vi "TEST LVOOP Plug Ins - Solution.vi"(8 "error in (no error)":errorcluster, 10 "Queue Name":string="Main") -> (0 "error out":errorcluster)   [LabVIEW 2011]
doc: "This is the solution that for the LVOOP Plug Ins exercise. It illustrates the power and flexibility of LVOOP plug ins.\n\nAAL 9/09"
uses:
  Report Class/Report.lvclass
  Shared/QDMH Poly VIs/QDMH POLY Enqueue String.vi
  Shared/QDMH Poly VIs/QDMH POLY Enqueue Strings.vi
panel:
  in  "Get Plug Ins":bool
  in  "File Name (no extension)":string
  in  "Header":string
  in  "Save to File":bool
  in  "Available Plug Ins":u16(ring) items=["TXT Report", "XML Report"]
  out "Message Display":string
  in  "Cancel":bool
  in  "OK":bool
  # "You must specify file name above."
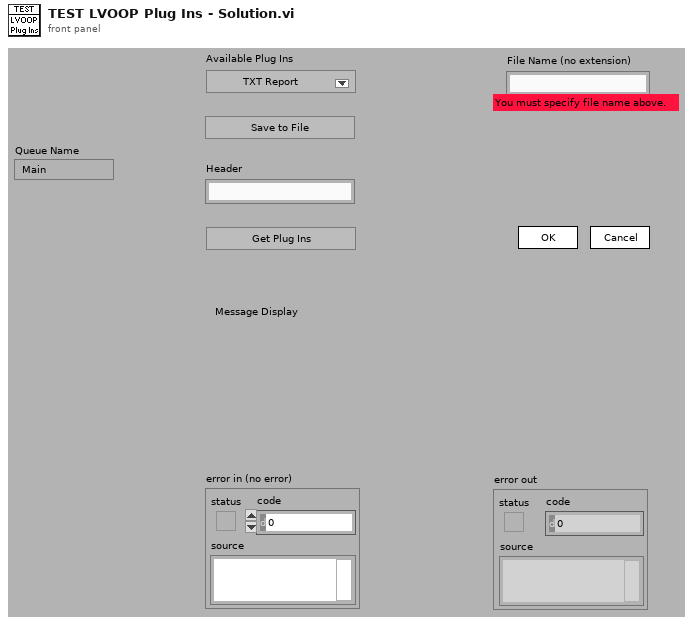
[diagram p1: front panel]
types:
  T1 = cluster{"Operator Name":string, "Current VI's Path":path, "Queue Names":string[], "# VIs Launched":i32, "Report Objects":refnum<class "Report.lvclass">[], "Selected Plug In":i32, "Current VI's Directory":path}
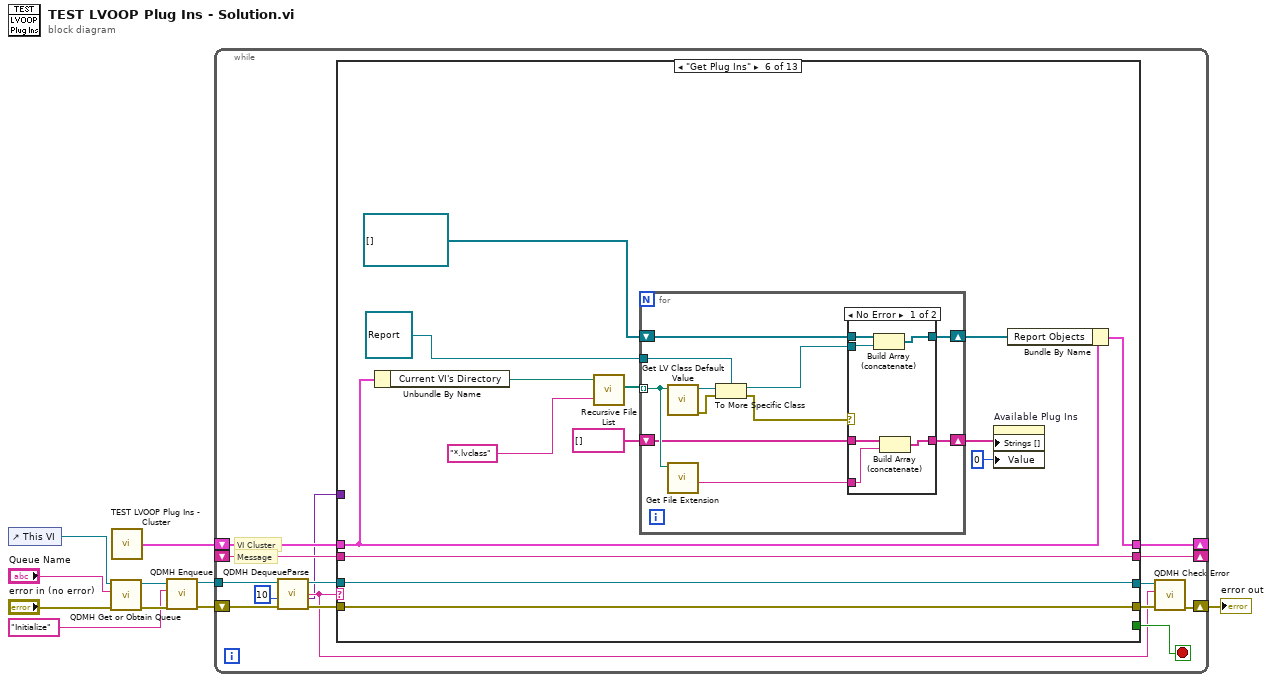
[diagram p0: block diagram]
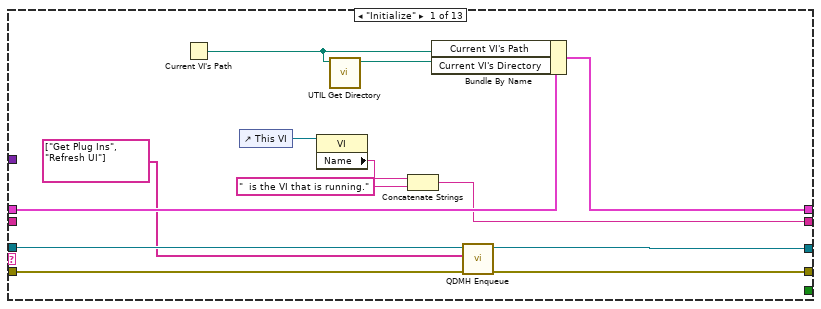
[diagram p2: hidden frame]
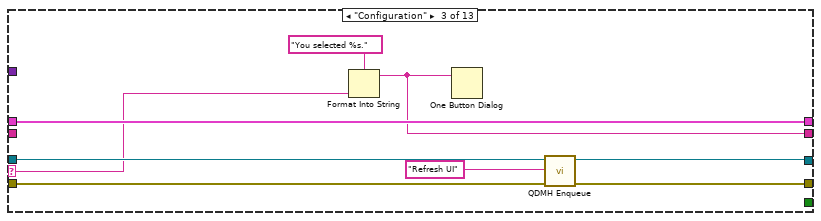
[diagram p4: hidden frame]
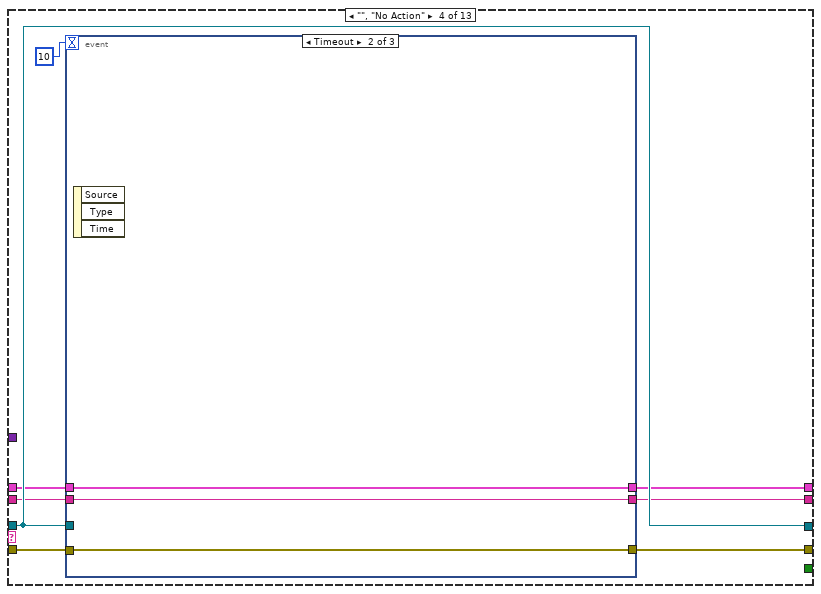
[diagram p5: hidden frame]
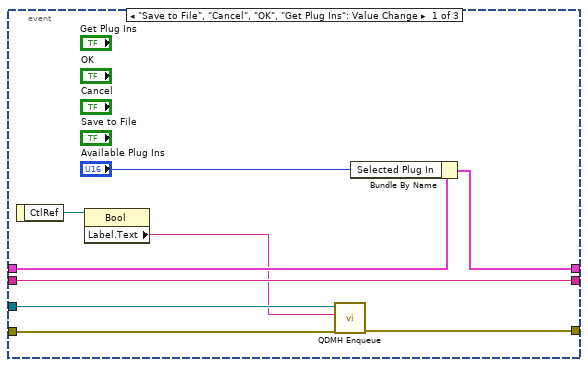
[diagram p6: hidden frame]
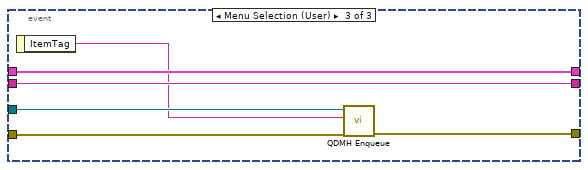
[diagram p7: hidden frame]
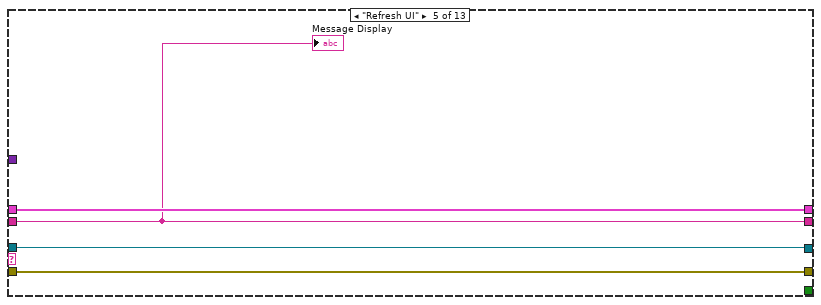
[diagram p8: hidden frame]
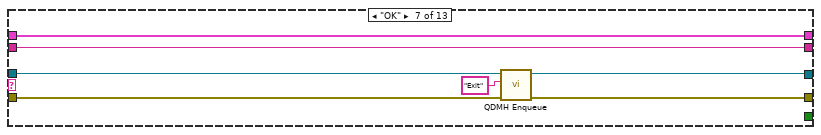
[diagram p10: hidden frame]
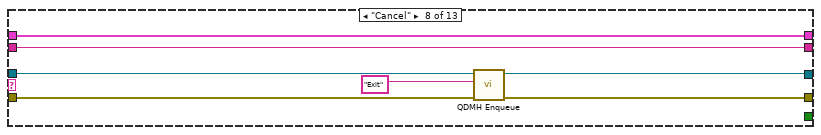
[diagram p11: hidden frame]
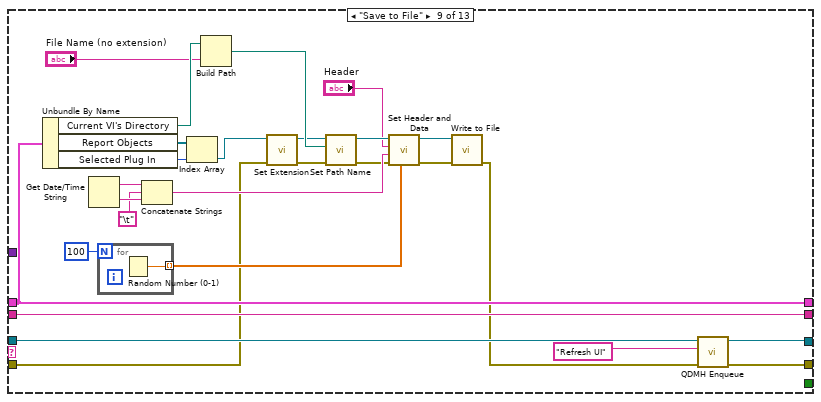
[diagram p12: hidden frame]
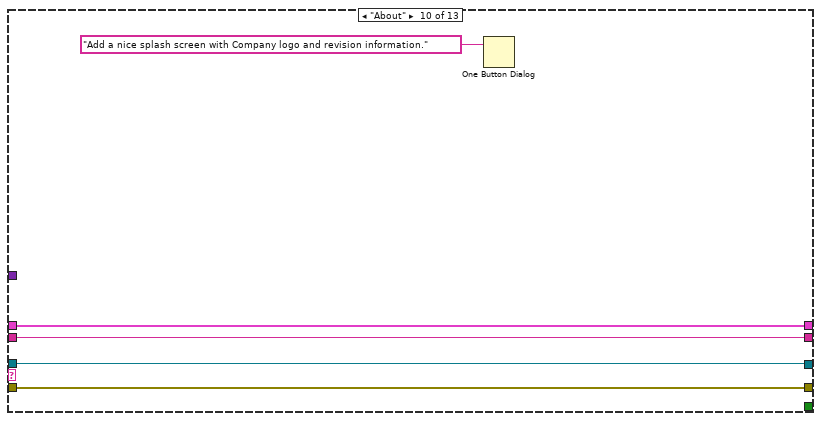
[diagram p13: hidden frame]
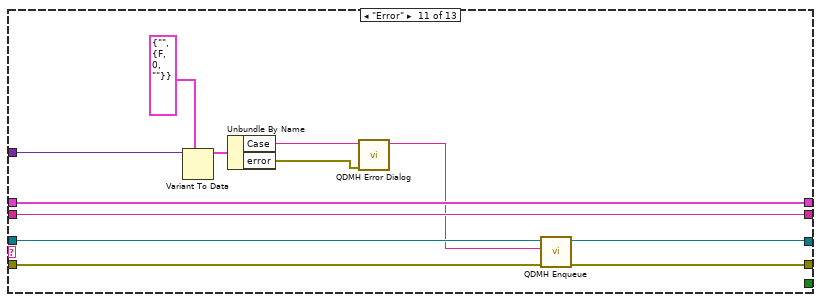
[diagram p14: hidden frame]
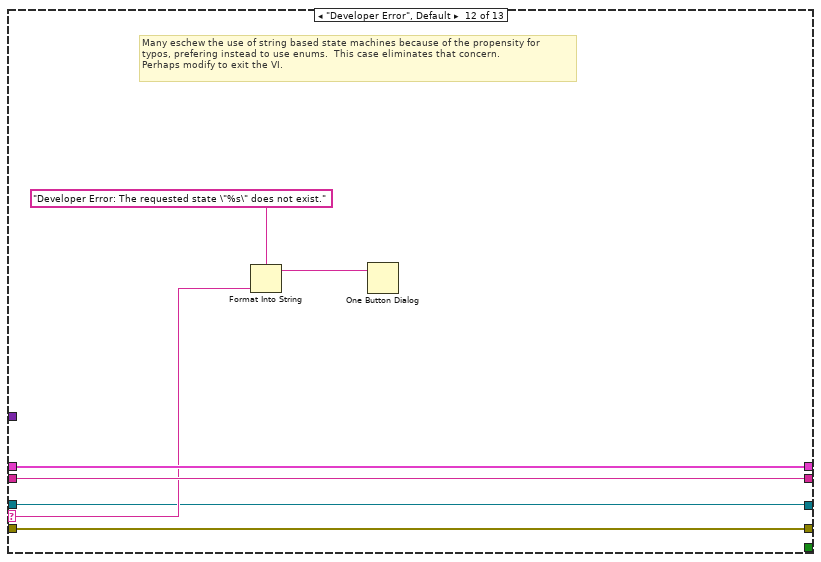
[diagram p15: hidden frame]
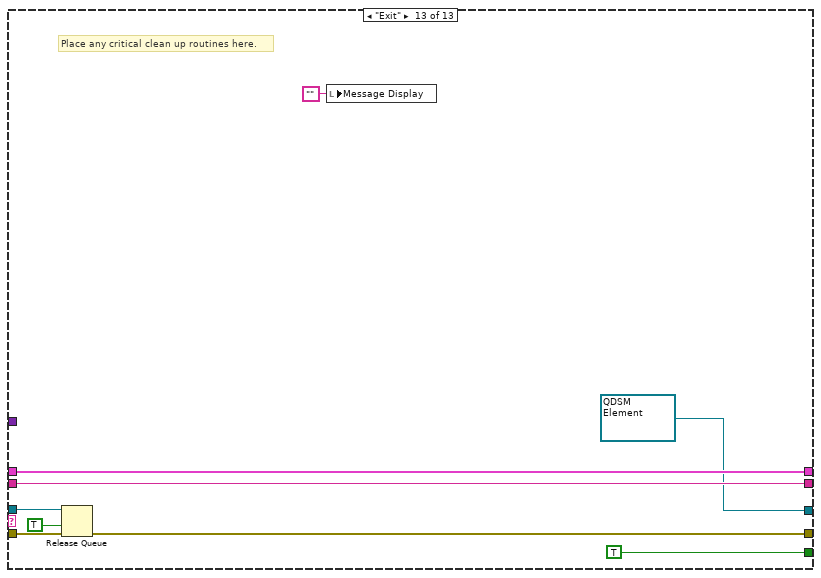
[diagram p16: hidden frame]
diagram:
  n1 = control-ref of="This VI"() -> (w2:refnum<vi>)
  n2 = call "QDMH Get or Obtain Queue.vi"("error in (no error)"="error in (no error)", "Queue Name"="Queue Name", "VI Refnum"=w2) -> ("error out"=w6:errorcluster, "queue out"=w9:refnum<queue>)  [unwired: 7 out]
  n3 = call "TEST LVOOP Plug Ins - Cluster.vi"() -> ("Cluster"=w8:T1)
  n4 = call-poly "QDMH Enqueue.vi"("error in (no error)"=w6, "State"="Initialize" ("element"), "queue"=w9) -> ("error out"=w7:errorcluster, "queue out"=w10:refnum<queue>)  [unwired: 7 in]
  n5 = while {
    tunnel: w10 -> [w21]
    shift-left: w8 -> [w22]
    shift-right: [w23] -> _
    shift-left: _ -> [w24]
    shift-right: [w14] -> _
    shift-right: [w12] -> w4
    shift-left: w7 -> [w17]
    stop <- w25 stop-if-true
    # "VI Cluster"
    # "Message"
    n6 = call "QDMH DequeueParse.vi"("error in (no error)"=w17, "Timeout"=10 ("ms timeout (-1)"), "queue"=w21) -> ("error out"=w18:errorcluster, "Variant Data"=w11:variant, "State"=w13:string, "queue out"=w19:refnum<queue>)  [unwired: 5 out]
    n7 = case shown="\"Get Plug Ins\"" w13 {
      selector: w13 -> [_ _ w47 _ _ _ _ _ _ _ _ w177 _]
      tunnel: w19 -> [w31 w39 w49 w59 w78 w83 w121 w128 w155 w157 w171 w174 w186]
      tunnel: [_ _ _ _ _ _ _ _ _ _ _ _ TRUE] -> w25
      tunnel: [w35 w42 w48 w52 w80 w95 w120 w127 w154 w161 w173 w180 w188] -> w14
      tunnel: w24 -> [_ w42 _ w53 w80 w95 w120 w127 w154 w161 w173 w180 w188]
      tunnel: [w37 w41 w51 w54 w81 w92 w119 w126 w152 w160 w172 w179 w183] -> w23
      tunnel: w22 -> [w38 w41 w51 w55 w81 w93 w119 w126 w152 w160 w172 w179 w183]
      tunnel: w18 -> [w32 w40 w46 w58 w79 w94 w118 w125 w132 w158 w170 w176 w185]
      tunnel: [w28 w40 w45 w57 w79 w94 w117 w124 w153 w158 w169 w176 w182] -> w16
      tunnel: [w27 w39 w43 w59 w78 w83 w115 w123 w130 w157 w168 w174 refnum<queue> refnum ("queue out")] -> w15
      tunnel: w11 -> [_ _ _ _ _ _ _ _ _ _ w163 _ _]
      frame "Initialize" {
        n8 = Current VI's Path() -> (path=w30:path)
        n9 = control-ref of="This VI"() -> (w34:refnum<vi>)
        n10 = property class="VI"(reference=w34) -> ("Name"=w33:string)  [unwired: 1 in, 2 out]
        n11 = call "UTIL Get Directory.vi"("Path In"=w30) -> ("Directory Out"=w29:path)  [unwired: 1 in, 9 out]
        n12 = Concatenate Strings(w33, "  is the VI that is running." ("string")) -> (w35:string)
        n13 = Bundle By Name(cluster=w38, "Current VI's Path"=w30, "Current VI's Directory"=w29) -> (w37:T1)
        n14 = call-poly "QDMH Enqueue.vi"("error in (no error)"=w32, "States"=string[] ["Get Plug Ins", "Refresh UI"], "queue"=w31) -> ("error out"=w28:errorcluster, "queue out"=w27:refnum<queue>)  [unwired: 7 in]
      }
      frame "Re-Initialize" {
        # "This case includes initialization functionality that may need to run again during the course of the VI"
      }
      frame "Configuration" {
        n15 = Format Into String(format string="You selected %s." ("Format String"), w47) -> (resulting string=w48:string)  [unwired: 2 in, 1 out]
        n16 = One Button Dialog(message=w48) -> ()  [unwired: 2 out]
        n17 = call-poly "QDMH Enqueue.vi"("error in (no error)"=w46, "State"="Refresh UI" ("New State"), "queue"=w49) -> ("error out"=w45:errorcluster, "queue out"=w43:refnum<queue>)  [unwired: 7 in]
      }
      frame "", "No Action" {
        n18 = event shown="[1] Timeout" {
          selector: _ -> [_ _ _]
          dyn-events: _ -> [_ _ _]
          timeout: 10 -> [_ _ _]
          tunnel: w59 -> [w67 _ w77]
          tunnel: [w66 w71 w75] -> w57
          tunnel: w58 -> [w65 w71 w76]
          tunnel: w55 -> [w63 w70 w74]
          tunnel: [w62 w70 w74] -> w54
          tunnel: w53 -> [w64 w69 w73]
          tunnel: [w64 w69 w73] -> w52
          event "Save to File", "Cancel", "OK", "Get Plug Ins": Value Change {
            n19 = event-data() -> ("CtlRef"=w68:refnum<vi>)  [unwired: 1 out]
            n20 = property class="Bool"(reference=w68) -> ("Label.Text"=w60:string)  [unwired: 1 in, 2 out]
            n21 = call-poly "QDMH Enqueue.vi"("error in (no error)"=w65, "State"=w60, "queue"=w67) -> ("error out"=w66:errorcluster)  [unwired: 7 in, 1 out]
            n22 = Bundle By Name(cluster=w63, "Selected Plug In"="Available Plug Ins") -> (w62:T1)
          }
          event Timeout {
            n23 = event-data() -> ()  [unwired: 4 out]
          }
          event Menu Selection (User) {
            n24 = event-data() -> ("ItemTag"=w72:string)  [unwired: 1 out]
            n25 = call-poly "QDMH Enqueue.vi"("error in (no error)"=w76, "State"=w72, "queue"=w77) -> ("error out"=w75:errorcluster)  [unwired: 7 in, 1 out]
          }
        }
      }
      frame "Refresh UI" {
        "Message Display" <- w80
      }
      frame "Get Plug Ins" {
        n26 = Unbundle By Name(w93) -> ("Current VI's Directory"=w82:path)
        n27 = call <vilib>:"Recursive File List.vi"("pattern"="*.lvclass", "Folder Path"=w82) -> ("All Files in Dir"=w89:path[])  [unwired: 2 in, 7 out]
        n28 = for {
          tunnel: w89 -> [w104] mode=indexing
          shift-right: [w100] -> w87
          shift-left: refnum<class "Report.lvclass">[] [] -> [w101]
          shift-right: [w102] -> w86
          shift-left: string[] [] -> [w103]
          tunnel: refnum<class "Report.lvclass"> refnum ("Report.lvclass") -> [w99]
          n29 = call <vilib>:"Get LV Class Default Value.vi"("class path"=w104) -> ("error out"=w106:errorcluster, "object"=w105:refnum<class>)  [unwired: 1 in, 8 out]
          n30 = call <vilib>:"Get File Extension.vi"("file"=w104) -> ("filename without extension"=w97:string)  [unwired: 1 in, 9 out]
          n31 = To More Specific Class(target class=w99, reference=w105, error in=w106) -> (specific class reference=w98:refnum<class "Report.lvclass">, error out=w96:errorcluster)
          n32 = case shown="No Error" w96 {
            tunnel: w101 -> [w109 w114]
            tunnel: [w108 w114] -> w100
            tunnel: w103 -> [w112 w113]
            tunnel: [w111 w113] -> w102
            tunnel: w97 -> [w110 _]
            tunnel: w98 -> [w107 _]
            frame No Error {
              n33 = Build Array (concatenate)(w109, w107) -> (w108:refnum<class "Report.lvclass">[])
              n34 = Build Array (concatenate)(w112, w110) -> (w111:string[])
            }
            frame Error {
            }
          }
        }
        n35 = property on="Available Plug Ins" class="Ring (strict)"("Strings []"=w86, "Value"=0) -> ()  [unwired: 2 in, 2 out]
        n36 = Bundle By Name(cluster=w93, "Report Objects"=w87) -> (w92:T1)
      }
      frame "OK" {
        n37 = call-poly "QDMH Enqueue.vi"("error in (no error)"=w118, "State"="Exit" ("New State"), "queue"=w121) -> ("error out"=w117:errorcluster, "queue out"=w115:refnum<queue>)  [unwired: 7 in]
      }
      frame "Cancel" {
        n38 = call-poly "QDMH Enqueue.vi"("error in (no error)"=w125, "State"="Exit" ("New State"), "queue"=w128) -> ("error out"=w124:errorcluster, "queue out"=w123:refnum<queue>)  [unwired: 7 in]
      }
      frame "Save to File" {
        n39 = Unbundle By Name(w152) -> ("Current VI's Directory"=w138:path, "Report Objects"=w150:refnum<class "Report.lvclass">[], "Selected Plug In"=w151:i32)
        n40 = Get Date/Time String() -> (date string=w145:string, time string=w147:string)  [unwired: 3 out]
        n41 = for {
          N: 100 -> [_]
          tunnel: [w156] -> w142 mode=indexing
          n42 = Random Number (0-1)() -> (number: 0 to 1=w156:dbl)
        }
        n43 = Concatenate Strings(w145, "\t", w147) -> (w144:string)
        n44 = Index Array(array=w150, index=w151) -> (element=w133:refnum<class "Report.lvclass">)
        n45 = Build Path(base path=w138, name or relative path="File Name (no extension)") -> (appended path=w136:path)
        n46 = call-dynamic "Set Extension.vi"("error in (no error)"=w132, "Report"=w133) -> ("error out"=w134:errorcluster, "Report out"=w135:refnum<class "Report.lvclass">)  [unwired: 8 out]
        n47 = call-dynamic "Set Path Name.vi"("error in (no error)"=w134, "Path"=w136, "Report"=w135) -> ("error out"=w140:errorcluster, "Report out"=w149:refnum<class "Report.lvclass">)  [unwired: 7 out]
        n48 = call-dynamic "Set Header and Data.vi"("Data Array"=w142, "error in (no error)"=w140, "Data & Time String"=w144, "Header"="Header", "Report"=w149) -> ("error out"=w139:errorcluster, "Report out"=w141:refnum<class "Report.lvclass">)  [unwired: 5 out]
        n49 = call-dynamic "Write to File.vi"("error in (no error)"=w139, "Report"=w141) -> ("error out"=w131:errorcluster)  [unwired: 9 out]
        n50 = call-poly "QDMH Enqueue.vi"("error in (no error)"=w131, "State"="Refresh UI" ("New State"), "queue"=w155) -> ("error out"=w153:errorcluster, "queue out"=w130:refnum<queue>)  [unwired: 7 in]
      }
      frame "About" {
        n51 = One Button Dialog(message="Add a nice splash screen with Company logo and revision information.") -> ()  [unwired: 2 out]
      }
      frame "Error" {
        n52 = Variant To Data(type=cluster{"Case":string, "error":errorcluster} {"Case"="", "error"={"status"=FALSE, "code"=0, "source"=""}} ("QDSM Element"), Variant=w163) -> (data=w166:cluster{"Case":string, "error":errorcluster})  [unwired: 1 in, 1 out]
        n53 = Unbundle By Name(w166) -> ("Case"=w165:string, "error"=w164:errorcluster)
        n54 = call "QDMH Error Dialog.vi"("error"=w164, "Case Error Occured"=w165) -> ("Case to Execute"=w162:string)  [unwired: 9 out]
        n55 = call-poly "QDMH Enqueue.vi"("error in (no error)"=w170, "State"=w162, "queue"=w171) -> ("error out"=w169:errorcluster, "queue out"=w168:refnum<queue>)  [unwired: 7 in]
      }
      frame "Developer Error", Default {
        # "Many eschew the use of string based state machines because of the propensity for\ntypos, prefering instead to use enums.  This case eliminates that concern.\nPerhaps modify to exit the VI."
        n56 = Format Into String(format string="Developer Error: The requested state \"%s\" does not exist." ("message"), w177) -> (resulting string=w175:string)  [unwired: 2 in, 1 out]
        n57 = One Button Dialog(message=w175) -> ()  [unwired: 2 out]
      }
      frame "Exit" {
        # "Place any critical clean up routines here."
        n58 = Release Queue(queue=w186, force destroy? (F)=TRUE, error in (no error)=w185) -> (error out=w182:errorcluster)  [unwired: 2 out]
        n59 = local write "Message Display"("") -> ()
      }
    }
    n60 = call "QDMH Check Error.vi"("error in (no error)"=w16, "Case"=w13, "queue"=w15) -> ("error out"=w12:errorcluster)  [unwired: 7 in, 1 out]
  }
  "error out" <- w4
